vi "ADCP_Get_Packet_Info_From_Raw_Packet.vi"(8 "error in (no error)":errorcluster, 10 "Raw Packet":u8[](array[numeric]), 11 "ADCP in":refnum<class "ADCP.lvclass">) -> (0 "error out":errorcluster, 2 "Checksum Valid ?":bool, 3 "ADCP out":refnum<class "ADCP.lvclass">, 4 "Packet frame ID":u8, 5 "Packet Type":T1(ring), 6 "Packet node ID":u8, 7 "Packet_Priority":enum16{"LOW", "HIGH"}(ring))   [LabVIEW 2017, in "ADCP.lvclass"]
uses:
  ADCP.lvclass
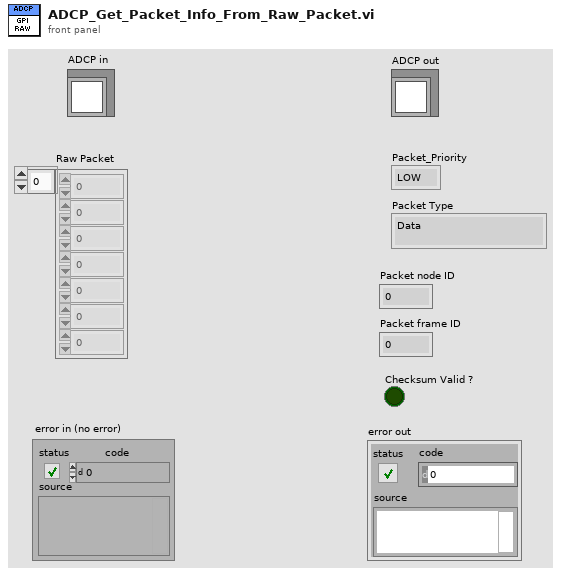
[diagram p1: front panel]
types:
  T1 = enum16{"Data", "Connection Management", "Remote Request", "Error and status", "INVALID"}
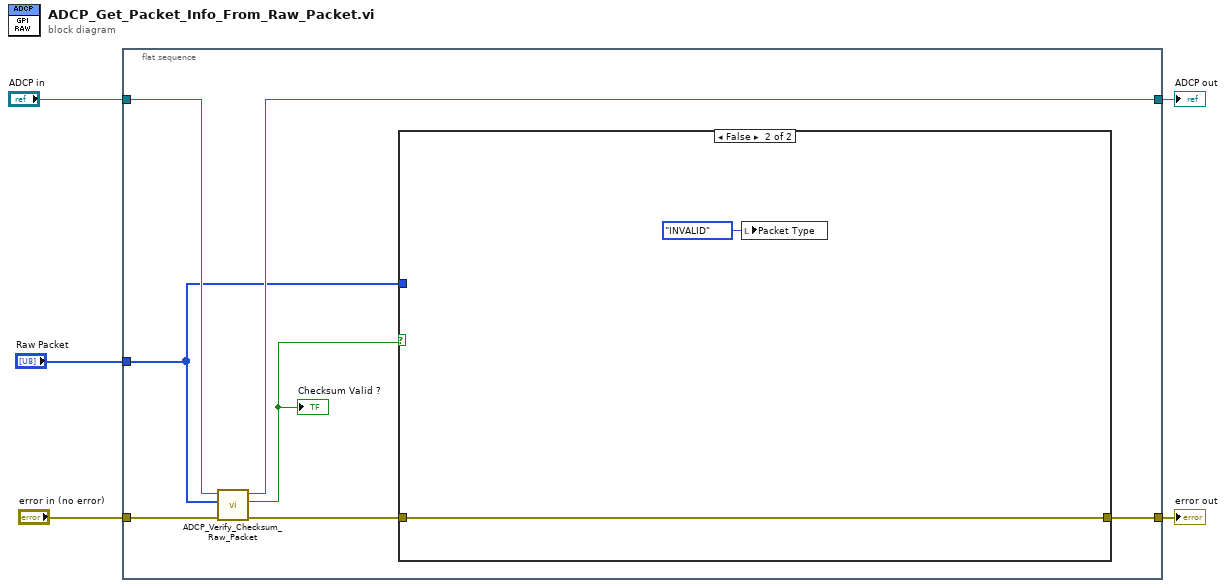
[diagram p0: block diagram]
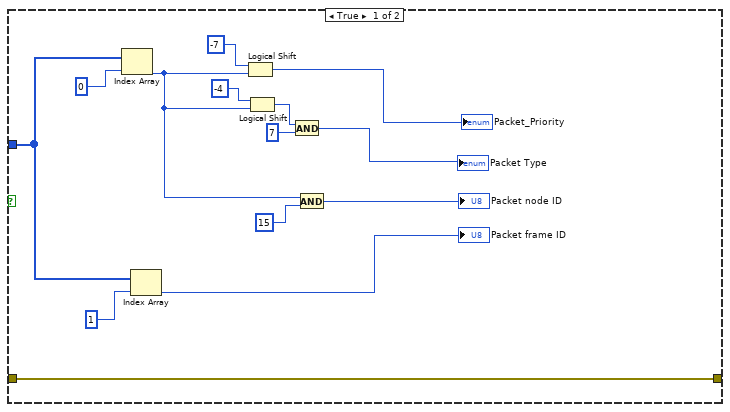
[diagram p2: hidden frame]
diagram:
  n1 = flat-sequence {
    tunnel: "ADCP in" -> [w11]
    tunnel: [w10] -> w4
    tunnel: "error in (no error)" -> [w12]
    tunnel: "Raw Packet" -> [w7]
    tunnel: [w6] -> w1
    frame #0 {
      n2 = call "ADCP_Verify_Checksum_Raw_Packet.vi"("error in (no error)"=w12, "Raw Packet"=w7, "ADCP in"=w11) -> ("error out"=w9:errorcluster, "Checksum Valid ?"=w8:bool, "ADCP out"=w10:refnum<class "ADCP.lvclass">)  [unwired: 6 in]
      "Checksum Valid ?" <- w8
      n3 = case shown="False" w8 {
        tunnel: w9 -> [w26 w28]
        tunnel: w7 -> [w15 _]
        tunnel: [w26 w28] -> w6
        frame True {
          n4 = Index Array(array=w15, index=0) -> (element=w18:u8)
          n5 = Index Array(array=w15, index=1) -> (element=→"Packet frame ID":u8)
          n6 = Logical Shift(y=i16 -7, x=w18) -> (x << y=→"Packet_Priority":u8)
          n7 = Logical Shift(y=i16 -4, x=w18) -> (x << y=w21:u8)
          n8 = And(x=w21, y=u8 7) -> (x .and. y?=→"Packet Type":u8)
          n9 = And(x=w18, y=u8 15) -> (x .and. y?=→"Packet node ID":u8)
        }
        frame False {
          n10 = local write "Packet Type"(T1."INVALID" ("Packet Type")) -> ()
        }
      }
    }
  }
  "ADCP out" <- w4
  "error out" <- w1
